vi "Create Sequence Call.vi"(4 "Group Number":i32=-1, 6 "Timeout ms (10000)":dbl=10000.0, 8 "error in (no error)":errorcluster, 9 "Target (\"\": Auto-assign)":string, 10 "Parameter Assignments":T2[](array[typedef]), 11 "Sequence File Path":path) -> (0 "error out":errorcluster, 3 "Sequence Call Ref":T1)   [LabVIEW 2020, in "NI_VS Sequence Execution Interface.lvlib"]
doc: "Specifies a sequence to execute using a file path you specify."
uses:
  <vilib>/NI VeriStand/Execution/SequenceExecutionInterface/NI_VS Sequence Execution Interface.lvlib
  <vilib>/NI VeriStand/Execution/SequenceExecutionInterface/Sequence Input Assignment Ref.ctl
  NationalInstruments.VeriStand.ClientAPI
  <vilib>/NI VeriStand/Execution/SequenceExecutionInterface/Sequence Call Ref.ctl
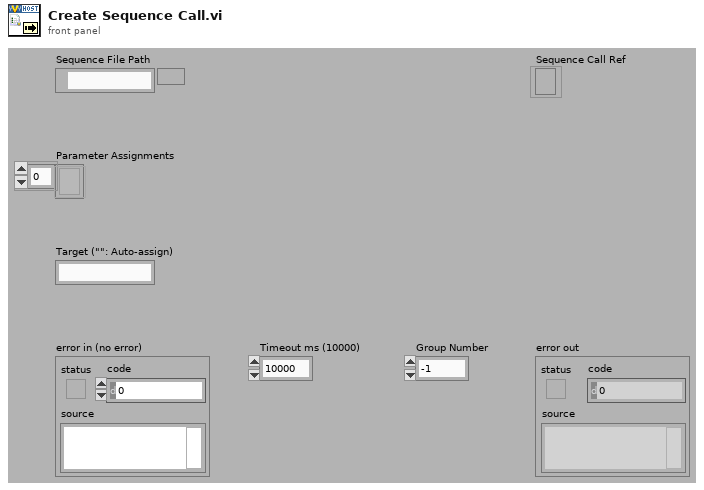
[diagram p1: front panel]
types:
  T1 = typedef "NI_VS Sequence Execution Interface.lvlib/Sequence Call Ref.ctl" = refnum<k24>
  T2 = typedef "NI_VS Sequence Execution Interface.lvlib/Sequence Input Assignment Ref.ctl" = refnum<k24>
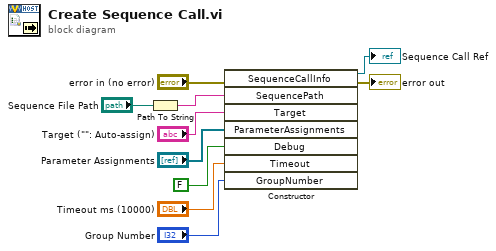
[diagram p0: block diagram]
diagram:
  n1 = Path To String(path="Sequence File Path") -> (string=w7:string)
  n2 = constructor class="SequenceCallInfo"(error in="error in (no error)", "SequencePath"=w7, "Target"="Target (\"\": Auto-assign)", "ParameterAssignments"="Parameter Assignments", "Debug"=FALSE, "Timeout"="Timeout ms (10000)", "GroupNumber"="Group Number") -> (reference out=→"Sequence Call Ref":refnum<k24>, error out=→"error out":errorcluster)  [unwired: 2 in, 7 out]
